vi "BRig_Host__Loop_Producer__UploadSettings_main__v2.vi"(9 "input_LoadSettings":bool, 10 "input_webdav_status":bool, 11 "session handle":T1) -> (0 "error out":errorcluster)   [LabVIEW 2014]
uses:
  <vilib>/WebDAVClient/Advanced/SessionHandle.ctl
  <vilib>/WebDAVClient/NI_WebDAV.lvlib
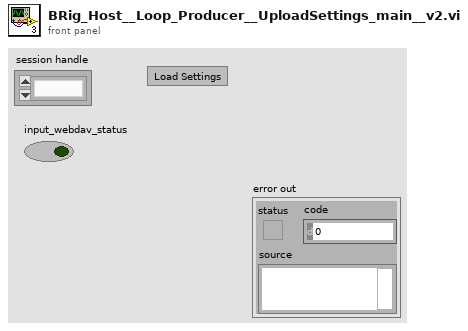
[diagram p1: front panel]
types:
  T1 = typedef "NI_WebDAV.lvlib/SessionHandle.ctl" = refnum<k1>
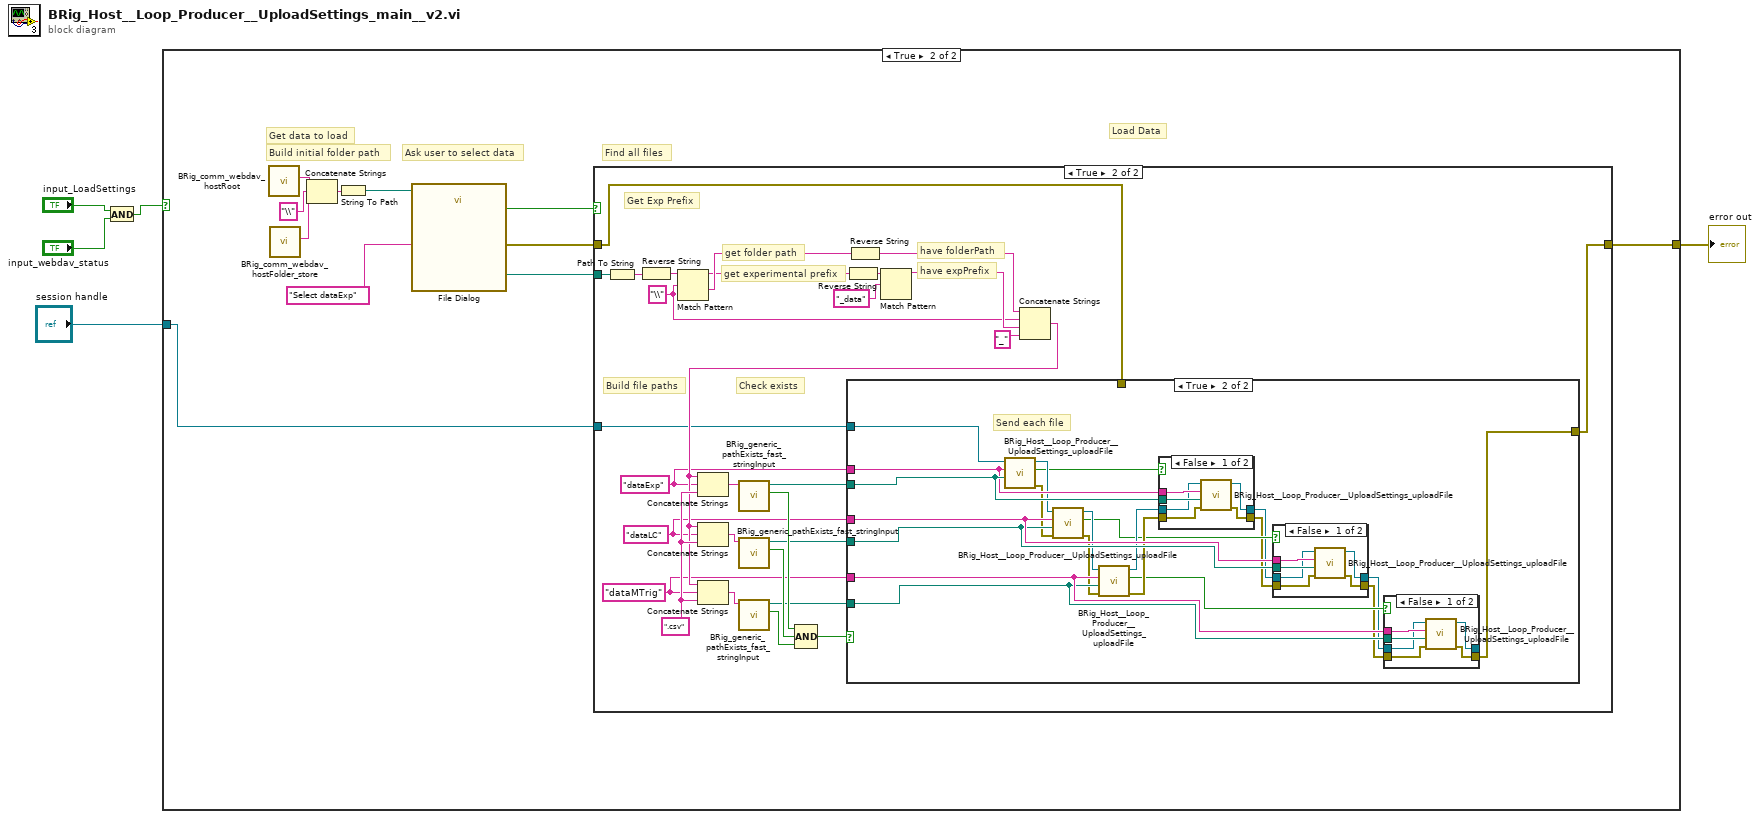
[diagram p0: block diagram]
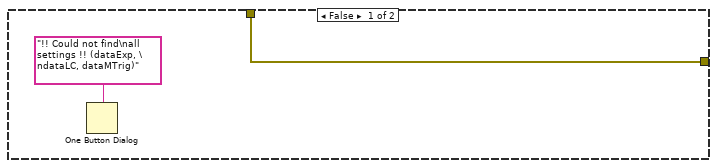
[diagram p4: hidden frame]
diagram:
  n1 = And(x="input_LoadSettings", y="input_webdav_status") -> (x .and. y?=w3:bool)
  n2 = case shown="True" w3 {
    tunnel: "session handle" -> [_ w8]
    tunnel: [_ w6] -> w1
    frame False {
    }
    frame True {
      # "Load Data"
      # "Find all files"
      # "Ask user to select data"
      # "Build initial folder path"
      # "Get data to load"
      n3 = call "BRig_comm_webdav_hostRoot.vi"() -> ("output_hostRoot"=w13:string)  [unwired: 11 in]
      n4 = call "BRig_comm_webdav_hostFolder_store.vi"() -> ("output_HostFolder"=w15:string)  [unwired: 11 in]
      n5 = Concatenate Strings(w13, "\\" ("string"), w15) -> (w16:string)
      n6 = String To Path(string=w16) -> (path=w12:path)
      n7 = call "File Dialog"("start path"=w12, "prompt"="Select dataExp") -> ("selected path"=w9:path, "exists"=w10:bool, "error out"=w7:errorcluster)  [unwired: 10 in, 1 out]
      n8 = case shown="True" w10 {
        tunnel: w9 -> [_ w36]
        tunnel: w8 -> [_ w20]
        tunnel: w7 -> [w17 w19]
        tunnel: [w17 w18] -> w6
        frame False {
        }
        frame True {
          w21 = "dataMTrig" ("regular expression")
          w22 = "dataLC" ("regular expression")
          w35 = ".csv" ("string")
          w23 = "dataExp" ("regular expression")
          w44 = "\\" ("regular expression")
          # "Check exists"
          # "Build file paths"
          # "get folder path"
          # "get experimental prefix"
          # "have expPrefix"
          # "have folderPath"
          # "Get Exp Prefix"
          n9 = Path To String(path=w36) -> (string=w37:string)
          n10 = Reverse String(1:w37) -> (0:w38:string)
          n11 = Match Pattern(string=w38, regular expression=w44) -> (before substring=w39:string, after substring=w42:string)  [unwired: 1 in, 2 out]
          n12 = Reverse String(1:w39) -> (0:w40:string)
          n13 = Reverse String(1:w42) -> (0:w43:string)
          n14 = Match Pattern(string=w40, regular expression="_data") -> (before substring=w45:string)  [unwired: 1 in, 3 out]
          n15 = Concatenate Strings(w43, w44, w45, "_" ("string")) -> (w34:string)
          n16 = Concatenate Strings(w34, w23, w35) -> (w33:string)
          n17 = Concatenate Strings(w34, w22, w35) -> (w32:string)
          n18 = Concatenate Strings(w34, w21, w35) -> (w31:string)
          n19 = call "BRig_generic_pathExists_fast_stringInput.vi"("input_filePath"=w33) -> ("output_Iexist"=w30:bool, "output_filePath"=w26:path)  [unwired: 8 in, 1 out]
          n20 = call "BRig_generic_pathExists_fast_stringInput.vi"("input_filePath"=w32) -> ("output_Iexist"=w29:bool, "output_filePath"=w25:path)  [unwired: 8 in, 1 out]
          n21 = call "BRig_generic_pathExists_fast_stringInput.vi"("input_filePath"=w31) -> ("output_Iexist"=w28:bool, "output_filePath"=w24:path)  [unwired: 8 in, 1 out]
          n22 = Compound Arithmetic op=AND(w30, w29, w28) -> (w27:bool)
          n23 = case shown="True" w27 {
            tunnel: w26 -> [_ w69]
            tunnel: w25 -> [_ w66]
            tunnel: w24 -> [_ w64]
            tunnel: w23 -> [_ w68]
            tunnel: w22 -> [_ w67]
            tunnel: w21 -> [_ w65]
            tunnel: w20 -> [_ w63]
            tunnel: w19 -> [w47 _]
            tunnel: [w47 w49] -> w18
            frame False {
              n24 = One Button Dialog(message="!! Could not find\nall settings !! (dataExp, \ndataLC, dataMTrig)") -> ()  [unwired: 1 in, 1 out]
            }
            frame True {
              # "Send each file"
              n25 = call "BRig_Host__Loop_Producer__UploadSettings_uploadFile.vi"("input_filePath_local"=w69, "dataName"=w68, "input_hSession"=w63) -> ("output_error"=w61:errorcluster, "output_Iexist"=w58:bool, "output_hSession"=w62:T1)  [unwired: 6 in]
              n26 = call "BRig_Host__Loop_Producer__UploadSettings_uploadFile.vi"("input_error"=w61, "input_filePath_local"=w66, "dataName"=w67, "input_hSession"=w62) -> ("output_error"=w59:errorcluster, "output_Iexist"=w55:bool, "output_hSession"=w60:T1)  [unwired: 5 in]
              n27 = call "BRig_Host__Loop_Producer__UploadSettings_uploadFile.vi"("input_error"=w59, "input_filePath_local"=w64, "dataName"=w65, "input_hSession"=w60) -> ("output_error"=w56:errorcluster, "output_Iexist"=w52:bool, "output_hSession"=w57:T1)  [unwired: 5 in]
              n28 = case shown="False" w58 {
                tunnel: w68 -> [w91 _]
                tunnel: w69 -> [w90 _]
                tunnel: w57 -> [w89 w93]
                tunnel: w56 -> [w88 w92]
                tunnel: [w87 w93] -> w54
                tunnel: [w86 w92] -> w53
                frame False {
                  n29 = call "BRig_Host__Loop_Producer__UploadSettings_uploadFile.vi"("input_error"=w88, "input_filePath_local"=w90, "dataName"=w91, "input_hSession"=w89) -> ("output_error"=w86:errorcluster, "output_hSession"=w87:T1)  [unwired: 5 in, 1 out]
                }
                frame True {
                }
              }
              n30 = case shown="False" w55 {
                tunnel: w67 -> [w83 _]
                tunnel: w66 -> [w82 _]
                tunnel: w54 -> [w81 w85]
                tunnel: w53 -> [w80 w84]
                tunnel: [w79 w85] -> w51
                tunnel: [w78 w84] -> w50
                frame False {
                  n31 = call "BRig_Host__Loop_Producer__UploadSettings_uploadFile.vi"("input_error"=w80, "input_filePath_local"=w82, "dataName"=w83, "input_hSession"=w81) -> ("output_error"=w78:errorcluster, "output_hSession"=w79:T1)  [unwired: 5 in, 1 out]
                }
                frame True {
                }
              }
              n32 = case shown="False" w52 {
                tunnel: w65 -> [w75 _]
                tunnel: w64 -> [w74 _]
                tunnel: w51 -> [w73 w77]
                tunnel: w50 -> [w72 w76]
                tunnel: [w71 w77] -> _
                tunnel: [w70 w76] -> w49
                frame False {
                  n33 = call "BRig_Host__Loop_Producer__UploadSettings_uploadFile.vi"("input_error"=w72, "input_filePath_local"=w74, "dataName"=w75, "input_hSession"=w73) -> ("output_error"=w70:errorcluster, "output_hSession"=w71:T1)  [unwired: 5 in, 1 out]
                }
                frame True {
                }
              }
            }
          }
        }
      }
    }
  }
  "error out" <- w1
